vi "NodeUI.vi"() -> ()   [LabVIEW 2013, in "NISE_CEF_Node.lvclass"]
doc: "UI that will be called when the node is selected."
uses:
  NISE_CEF_Node.lvclass
  NodeRef.ctl
  <vilib>/NI/AMC/Message Queue.ctl
  <vilib>/NI/AMC/Message.ctl
  <vilib>/NI/Tools/Keyed Array/KeyedArray.ctl
  UserEventRef.ctl
  Controls/EventCluster.ctl
  <vilib>/NI/AMC/Create Single Message.vi
  <vilib>/NI/AMC/Update Message Routing Info.vi
  <vilib>/NI/AMC/Send Message.vi
  <vilib>/NI/AMC/AMC.lvlib
  <vilib>/NI/Tools/Keyed Array/Tools_KeyedArray.lvlib
  NISE_CEF_TreeControl.lvlib
panel:
  out "Numeric":i32
  in  "user event":T1
  in  "main queue":T2
  in  "String":string
  in  "node ref":T3
  # "Default node UI\nNo UI has been created for this type of node."
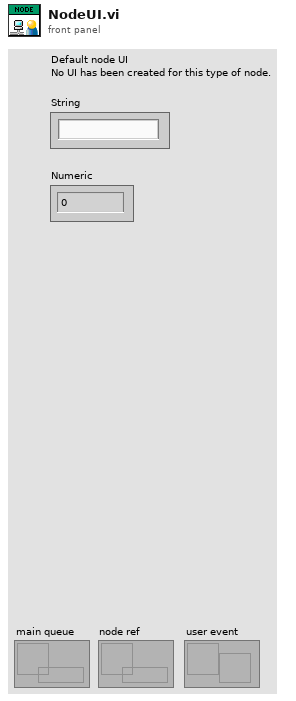
[diagram p1: front panel]
types:
  T1 = typedef "NISE_CEF_Node.lvclass/UserEventRef.ctl" = refnum<user-event>
  T2 = typedef "AMC.lvlib/Message Queue.ctl" = refnum<queue>
  T3 = typedef "NISE_CEF_Node.lvclass/NodeRef.ctl" = refnum<data-value>
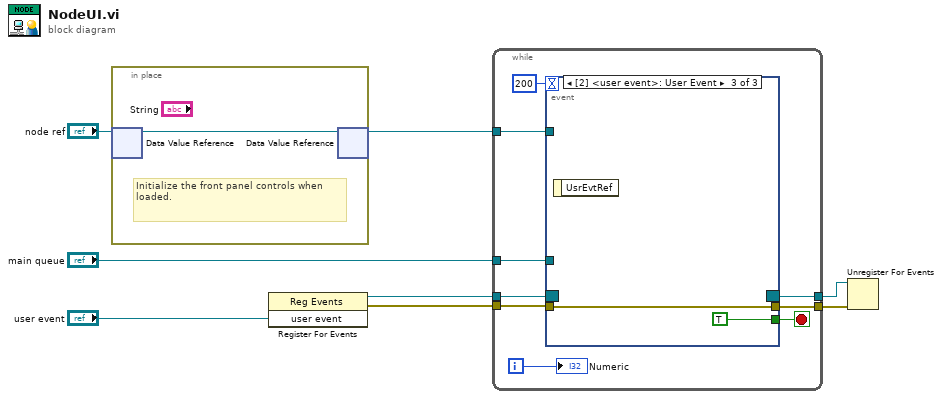
[diagram p0: block diagram]
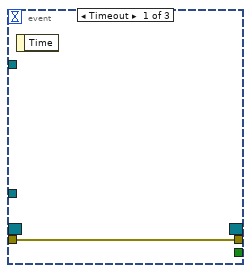
[diagram p2: hidden frame]
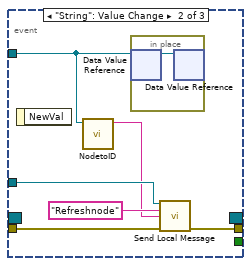
[diagram p3: hidden frame]
diagram:
  n1 = in-place {
    # "Initialize the front panel controls when loaded."
    n2 = in-place-dvr #1("node ref") -> (w9:refnum<class "NISE_CEF_Node.lvclass">)  [unwired: 1 out]
    n3 = in-place-dvr #1(w9) -> (w7:T3)  [unwired: 1 out]
  }
  n4 = register-events("user event") -> (reference out=w4:refnum<event-registration>, error out=w1:errorcluster)  [unwired: 2 in]
  n5 = while {
    tunnel: w7 -> [w18]
    tunnel: "main queue" -> [w17]
    tunnel: w4 -> [w15]
    tunnel: [w14] -> w3
    tunnel: [w12] -> w2
    tunnel: w1 -> [w11]
    i -> [w10]
    stop <- w13 stop-if-true
    n6 = event shown="[2] <user event>: User Event" {
      selector: w15 -> [_ _ _]
      dyn-events: [_ _ _] -> w14
      timeout: 200 -> [_ _ _]
      tunnel: w18 -> [_ w23 _]
      tunnel: w17 -> [_ w24 _]
      tunnel: [_ _ TRUE] -> w13
      tunnel: [w19 w21 w27] -> w12
      tunnel: w11 -> [w19 w20 w27]
      event Timeout {
        n7 = event-data() -> ()  [unwired: 1 in, 1 out]
      }
      event "String": Value Change {
        n8 = event-data() -> ()  [unwired: 1 in, 1 out]
        n9 = call "NodetoID.vi"("node ref"=w23) -> ("ID"=w22:string)  [unwired: 9 in, 1 out]
        n10 = in-place {
          n11 = in-place-dvr #2(w23) -> (w26:refnum<class "NISE_CEF_Node.lvclass">)  [unwired: 1 out]
          n12 = in-place-dvr #2(w26) -> ()  [unwired: 2 out]
        }
        n13 = call <vilib>:"Send Local Message.vi"("message queue in"=w24, "message name"="Refreshnode" ("Message Name"), "message value"=w22, "error in"=w20) -> ("error out"=w21:errorcluster)  [unwired: 9 in, 2 out]
      }
      event User Event {
        n14 = event-data() -> ()  [unwired: 1 in, 1 out]
      }
    }
    "Numeric" <- w10
  }
  n15 = Unregister For Events(event registration refnum=w3, error in=w2) -> ()  [unwired: 1 out]
